vi "Write Main App Inst Ref.vi"(8 "error in (no error)":errorcluster, 10 "Main App Inst Ref":refnum<vi>, 11 "Project in":refnum<class "Project.lvclass">) -> (0 "error out":errorcluster, 3 "Project out":refnum<class "Project.lvclass">)   [LabVIEW 2019, in "Panther Dashboard.lvlib" / "Project.lvclass"]
uses:
  Project.lvclass
  Project.lvclass/Project.ctl
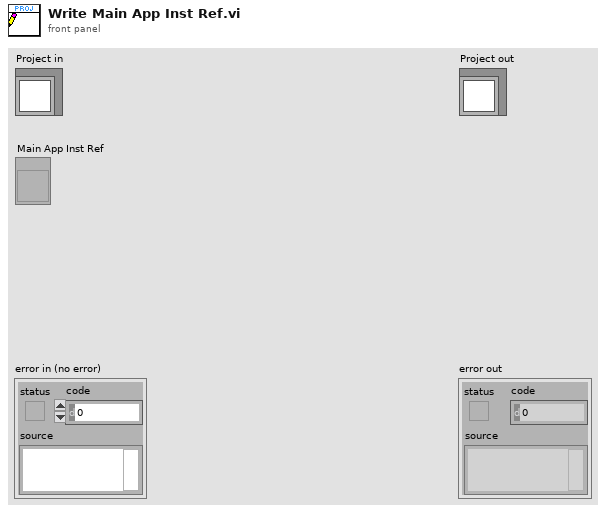
[diagram p1: front panel]
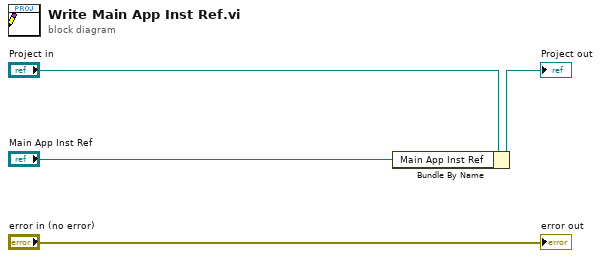
[diagram p0: block diagram]
diagram:
  n1 = Bundle By Name(cluster="Project in", "Main App Inst Ref"="Main App Inst Ref") -> (→"Project out":refnum<class "Project.lvclass">)
  "error out" <- "error in (no error)"
